vi "poc.ip.versal.vi"(0 "ip.reset":bool, 1 "TDATA":u64, 2 "TKEEP":u8, 3 "TUSER":bool, 4 "TVALID":bool, 5 "TLAST":bool) -> ()   [LabVIEW 2025]
uses:
  <vilib>/Platform/TimedLoop/XDataNode/timing_clust.ctl
  <vilib>/Platform/TimedLoop/XDataNode/nitl_modes.ctl
  <vilib>/Platform/TimedLoop/XDataNode/wakeup.ctl
  submodules/Market.Data.Common/fpga/my.network.data.stream.ctl
  submodules/Market.Data.Bats.Parser/fpga/poc.ip.debug.states.ctl
  submodules/Market.Data.Common/fpga/orderbook.command.ctl
  submodules/Market.Data.Common/fpga/orderbook.command.type.ctl
  submodules/Market.Data.Bats.Parser/fpga/poc.ip.axi.write.states.ctl
  <instrlib>/_niInstr/Network/Types/v1/IPv4 Address.ctl
  <instrlib>/_niInstr/Network/Types/v1/MAC Address.ctl
  Ethernet MAC - Custom/Ethernet MAC - Custom.lvclass
  axi_2_eth_raw.ctl
  <vilib>/rvi/DataTransferAndStorage/Container/Common/niFpgaContainerGetUniqueNameForEmu.vi
  <vilib>/rvi/DataTransferAndStorage/Container/Common/niFpgaContainerSetEmuInfo.vi
  <vilib>/rvi/eio/common/nirviEmuReportErrorAndStop.vi
  <vilib>/rvi/Emulation/niFpgaSctlEmulationGetInTimedLoop.vi
  <vilib>/rvi/Emulation/niFpgaEmulationReportErrorSimple.vi
  <vilib>/rvi/Emulation/niFpgaGetClockAttributes.vi
  <vilib>/rvi/Emulation/niFpgaCriticalErrorInLSC.vi
  <vilib>/rvi/Emulation/niFpgaEmulationIsFPGAContextNoSignature.vi
  <vilib>/rvi/errors/niFpgaSetErrorForExecOnDevCompSimple.vi
  <vilib>/rvi/FIFO/Fifo_Resource/nirvififoEmulationSetSize.vi
  <vilib>/rvi/FIFO/Fifo_Resource/nirviFifoEmulationQueueMgr.vi
  <instcachedir>/0/nirviFifoEmulationQueueMgr_E5CAEC123FF24DC58D834DCA3CDAA9B5.lvgen/nirviFifoEmulationQueueMgr_E5CAEC123FF24DC58D834DCA3CDAA9B5_002.vi
  <vilib>/Utility/error.llb/Clear Errors.vi
  <vilib>/rvi/FIFO/Fifo_Resource/nirvififoEmulationCreateLock.vi
  <vilib>/rvi/Emulation/niFpgaProcessEmulError.vi
  <vilib>/rvi/FIFO/Fifo_Resource/nirvififoEmulationObtainLock.vi
  <vilib>/rvi/FIFO/Fifo_Resource/nirvififoEmulationReleaseLock.vi
  <vilib>/rvi/occurrence/nirviWaitOnOccurrenceBase.vi
  <vilib>/rvi/errors/nirviReportUnexpectedCaseInternalError.vi
  <vilib>/rvi/errors/nirviReportUnexpectedCaseInternalError (U32).vi
  <vilib>/rvi/interface/RandomDataEmulation/nirviRandomDataMultiElementFPGAFIFO.vi
  <instcachedir>/0/nirviRandomDataMultiElementFPGAFIFO_BE2FF10D3D6E420AB0291A02835C249E.lvgen/nirviRandomDataMultiElementFPGAFIFO_BE2FF10D3D6E420AB0291A02835C249E_001.vi
  <vilib>/rvi/interface/RandomDataEmulation/niFpgaRandomDataHandleErrors.vi
  <instcachedir>/0/nirviFifoEmulationQueueMgr_E5CAEC123FF24DC58D834DCA3CDAA9B5.lvgen/nirviFifoEmulationQueueMgr_E5CAEC123FF24DC58D834DCA3CDAA9B5_004.vi
  <vilib>/rvi/DataTransferAndStorage/Container/Common/niFpgaContainerExecOnDevCompGetState.vi
  <vilib>/rvi/Memory/Memory_Emulation/niFpgaMemoryEmulationCacheClearOnFirstRun.vi
  <vilib>/rvi/Memory/Memory_Emulation/nirvimemoryEmulationManagerCache_MakeExclusive.vi
  <vilib>/rvi/Memory/Memory_Emulation/niFpgaMemoryEmulationValidateCache.vi
  <vilib>/rvi/Memory/Memory_Emulation/nirvimemoryEmulationManagerCache_InsertValue.vi
  <vilib>/rvi/Memory/Memory_Emulation/nirvimemoryEmulationManagerCache_ReleaseExclusive.vi
  <vilib>/rvi/Memory/Memory_Emulation/nirvimemoryEmulationManagerCache_GetValue.vi
  <vilib>/rvi/Memory/Memory_Emulation/nirvimemoryEmulationManagerCache_SetValue.vi
  <instcachedir>/0/nirviFifoEmulationQueueMgr_E5CAEC123FF24DC58D834DCA3CDAA9B5.lvgen/nirviFifoEmulationQueueMgr_E5CAEC123FF24DC58D834DCA3CDAA9B5_005.vi
  <vilib>/rvi/FIFO/Fifo_Resource/nirvififoEmulationDetermineInputValidOut.vi
  <vilib>/eio/utilities/niEioResolveVilibRelativePath.vi
  <instcachedir>/0/nirviFifoEmulationQueueMgr_E5CAEC123FF24DC58D834DCA3CDAA9B5.lvgen/nirviFifoEmulationQueueMgr_E5CAEC123FF24DC58D834DCA3CDAA9B5_003.vi
  <vilib>/rvi/Emulation/niFpgaSctlEmulationResourceMgr.vi
  <instrlib>/_niInstr/Network/IPv4/Data Stream/v1/Read IPv4 Header.vi
  <instrlib>/_niInstr/Network/IPv4/UDP/Data Stream/v1/Read End of Bad Frame.vi
  <instrlib>/_niInstr/Network/IPv4/UDP/Data Stream/v1/Read End of Good Frame.vi
  <instrlib>/_niInstr/Network/IPv4/UDP/Data Stream/v1/Read Data Stream.vi
  <vilib>/Platform/TimedLoop/XDataNode/XDataNode.xnode
  <vilib>/rvi/LocalResourceManager/LocalResourceManager.xnode
  <vilib>/rvi/DataTransferAndStorage/Container/XNode/niFpgaContainer.xnode
  <vilib>/rvi/FIFO/Fifo_Resource/nirvififoEmulationRead.vi
  <vilib>/rvi/interface/RandomDataEmulation/nirviRandomDataFpgaMultiElementTemplate.vi
  <vilib>/rvi/DataTransferAndStorage/Register/Emulation/niFpgaRegisterEmulationRefIn.vi
  <vilib>/rvi/FIFO/Fifo_Resource/niFpgaFifoEmulationRefIn.vi
  <vilib>/rvi/Memory/Memory_Emulation/niFpgaMemoryEmulationRefIn.vi
  <vilib>/rvi/FIFO/Fifo_Resource/nirvififoEmulationWrite.vi
  <vilib>/Platform/TimedLoop/XDataNode/XDNodeRunTimeDep.lvlib
  submodules/Market.Data.Common/fpga/fpganow.common.fpga.lvlib
  <instrlib>/_niInstr/Network/IPv4/UDP/Data Stream/v1/niInstr IPv4 UDP Data Stream v1.lvclass
  <instrlib>/_niInstr/Network/Ethernet/Utility/v1/FPGA/niInstr Ethernet Utilities FPGA v1.lvlib
  <instrlib>/_niInstr/Network/IPv4/FPGA/v1/niInstr IPv4 FPGA v1.lvlib
  <instrlib>/_niInstr/Network/IPv4/UDP/FPGA/v1/niInstr IPv4 UDP FPGA v1.lvlib
  <instrlib>/_niInstr/Network/Types/v1/niInstr Network Types v1.lvlib
  <instrlib>/_niInstr/Network/IPv4/Data Stream/v1/niInstr IPv4 Data Stream v1.lvclass
panel:
  in  "DEBUG.TREADY":bool
  in  "CMD.TREADY":bool
  in  "MDEBUG.TREADY":bool
  out "MDEBUG.TLAST":bool
  out "MDEBUG.TVALID":bool
  out "MDEBUG.TKEEP":u8
  out "MDEBUG.TDATA":u64
  out "CMD.TKEEP":u8
  out "CMD.TDATA":u64
  out "CMD.TLAST":bool
  out "CMD.TVALID":bool
  out "DEBUG.TLAST":bool
  out "DEBUG.TVALID":bool
  out "DEBUG.TKEEP":u8
  out "DEBUG.TDATA":u64
  # "This VI will be IP Exported"
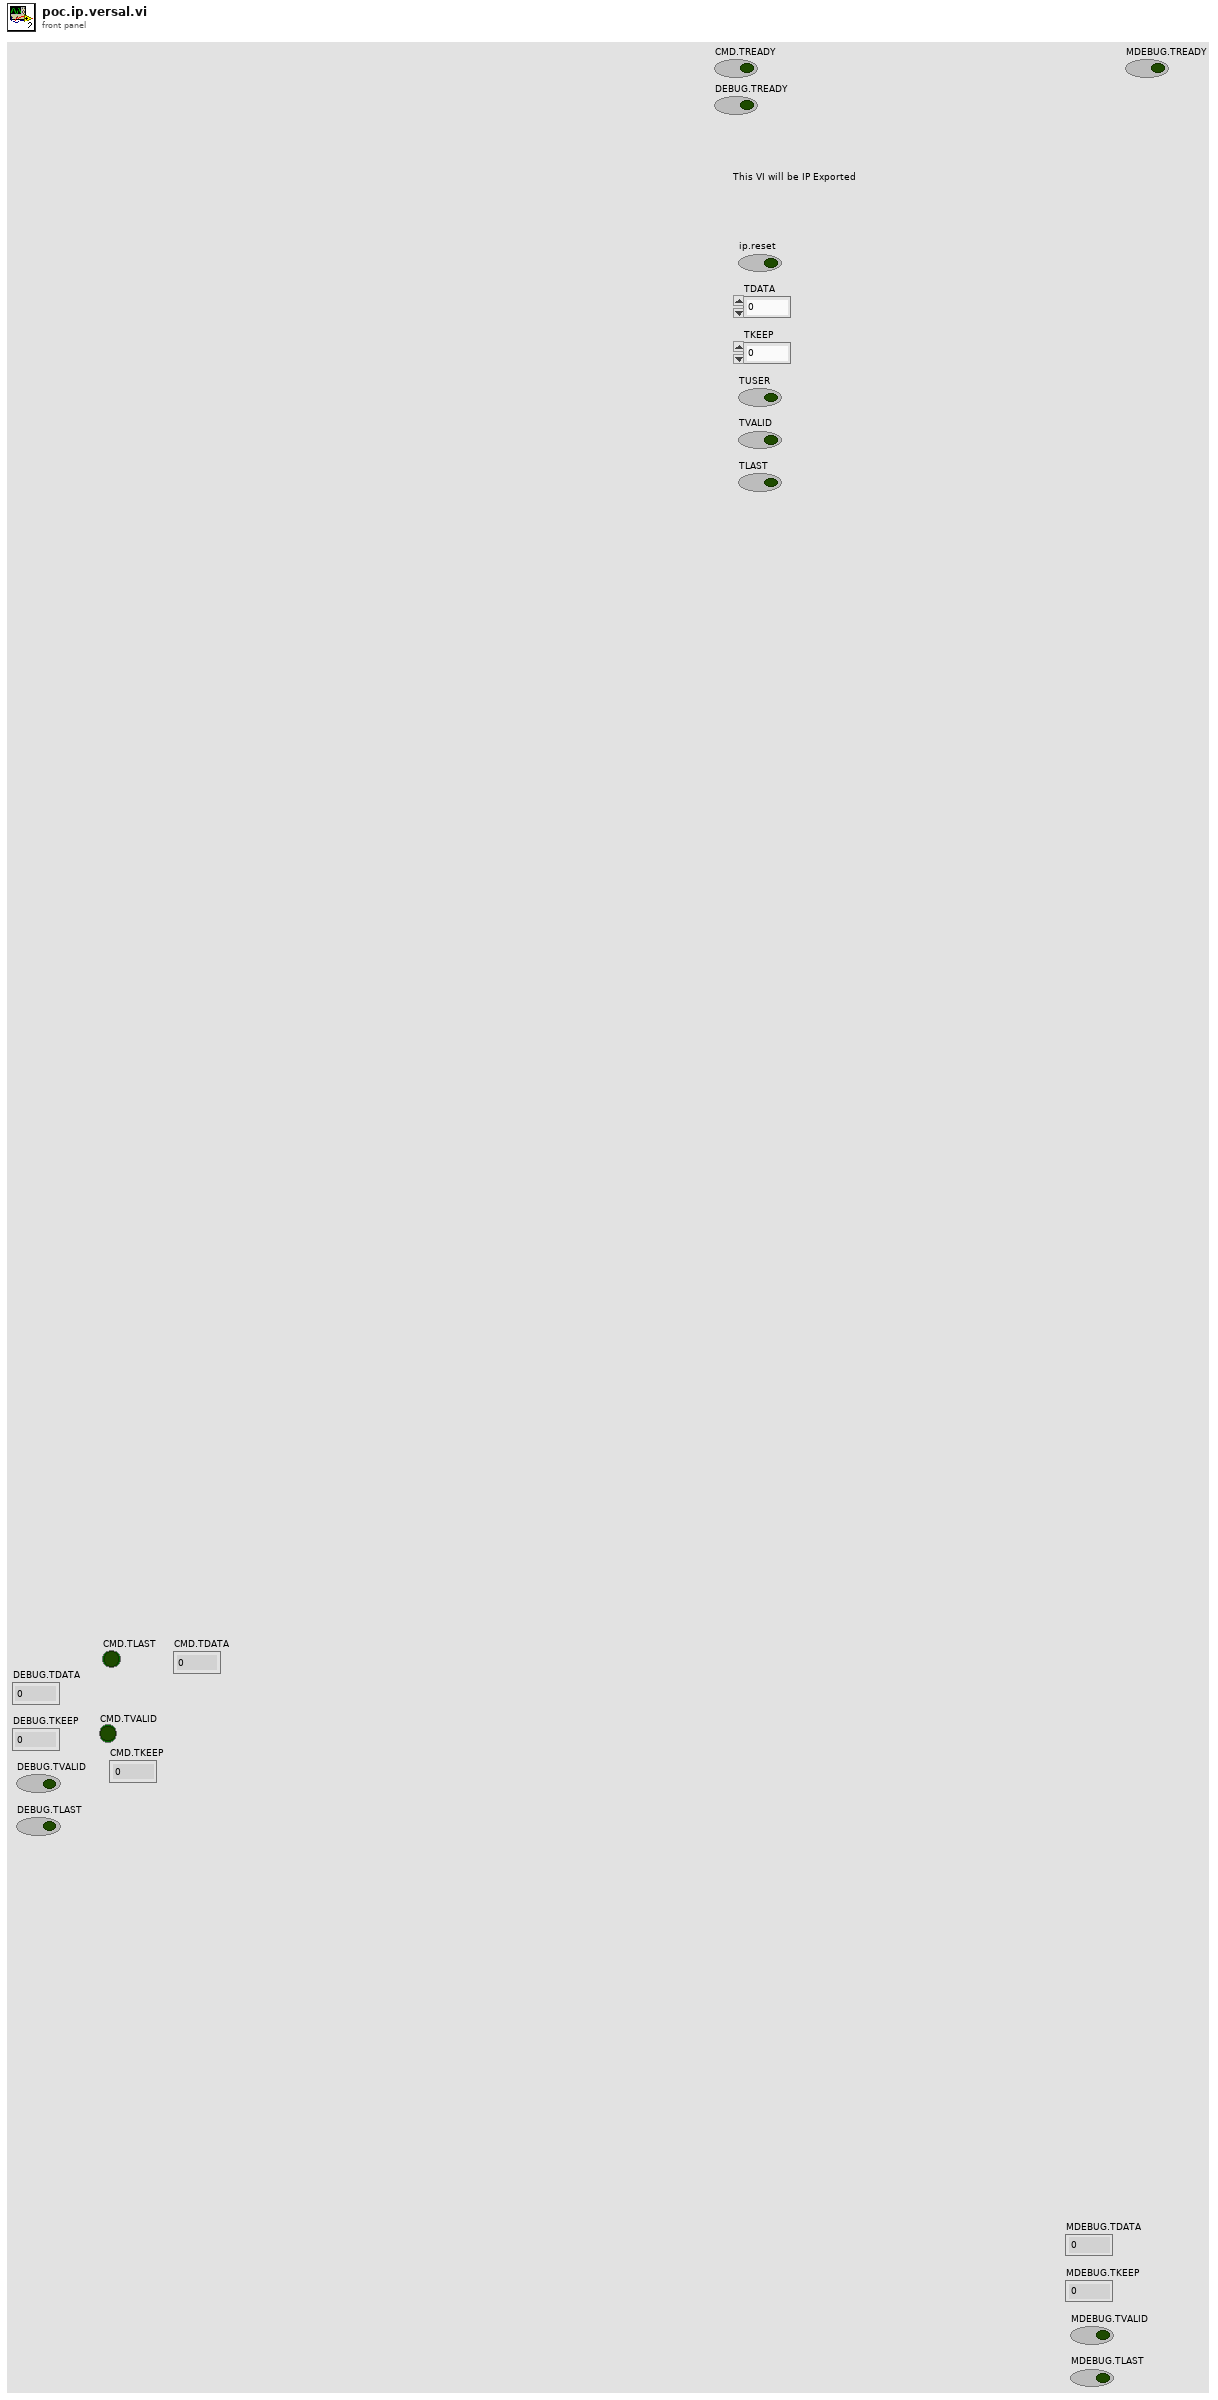
[diagram p1: front panel]
types:
  T1 = typedef "XDNodeRunTimeDep.lvlib/timing_clust.ctl" = cluster{"Expected End [f-1]":u64, "Actual End [f-1]":u64, "Finished Late? [f-1]":bool, "Expected End [i-1]":u64, "Actual End [i-1]":u64, "Finished Late? [i-1]":bool, "Expected Start [i]":u64, "Actual Start [i]":u64, "Expected Start [f]":u64, "Actual Start [f]":u64, "Source Name":string, "Structure Name":string, "Period":i64, "Deadline":i64, "Offset":i64, "Start":i64, "Priority":i32, "Timeout":i32, "Mode":T2, "Wakeup Reason":T3, "Error":errorcluster, "Source Type":string, "Secondary Source Type":string, "Global End Time":u64, "Global Start Time":u64, "Frame Duration":u64, "Iteration Duration":u64, "Assigned CPU":i32, "I/O Scan Engine Mode":u32}
  T2 = typedef "XDNodeRunTimeDep.lvlib/nitl_modes.ctl" = enum32{"No Change", "Process missed periods, maintain original phase", "Discard missed periods, maintain original phase", "Process missed periods, ignore original phase", "Discard missed periods, ignore original phase"}
  T3 = typedef "XDNodeRunTimeDep.lvlib/wakeup.ctl" = enum32{"Normal", "Aborted", "Asynchronous wakeup", "Timing source error", "Timed loop error", "Timeout"}
  T4 = typedef "niInstr Network Types v1.lvlib/MAC Address.ctl" = u8[]
  T5 = typedef "niInstr Network Types v1.lvlib/IPv4 Address.ctl" = u8[]
  T6 = typedef "my.network.data.stream.ctl" = cluster{"data":u8[], "data valid":bool, "byte enables":bool[], "eof.good":bool, "eof.bad":bool, "Timestamp":u64}
  T7 = cluster{"TDATA":u64, "TKEEP":u8, "TVALID":bool, "TLAST":bool, "TUSER":bool}
  T8 = cluster{"data valid":bool, "end.of.frame":bool, "start.of.frame":bool, "data":u64, "byte enables":u8}
  T9 = typedef "axi_2_eth_raw.ctl" = cluster{"data valid":bool, "end.of.frame":bool, "start.of.frame":bool, "data":u64, "byte enables":u8}
  T10 = typedef "niInstr IPv4 FPGA v1.lvlib/IPv4 Header.ctl" = cluster{"Version":fxp<+,4,4>, "IHL":fxp<+,4,4>, "DSCP":fxp<+,6,6>, "ECN":fxp<+,2,2>, "Total Length":u16, "Identification":u16, "Flags":fxp<+,3,3>, "Fragment Offset":fxp<+,13,13>, "Time To Live":u8, "Protocol":T11, "Header Checksum":u16, "Source IP":u8[], "Dest IP":u8[]}
  T11 = typedef "niInstr IPv4 FPGA v1.lvlib/IPv4 Protocols.ctl" = u8
  T12 = typedef "niInstr Ethernet Utilities FPGA v1.lvlib/Network Data Stream.ctl" = cluster{"data":u8[], "data valid":bool, "byte enables":bool[]}
  T13 = typedef "poc.ip.axi.write.states.ctl" = enum16{"Wait", "Collect"}
  T14 = typedef "poc.ip.debug.states.ctl" = enum16{"Wait", "Write.Data"}
  T15 = typedef "fpganow.common.fpga.lvlib/orderbook.command.ctl" = cluster{"type":T16, "side":u8, "orderId ":u64, "quantity":u32, "symbol":u64, "price":u64, "executed.qty":u32, "canceled.qty":u32, "remaining.qty":u32, "seconds":u64, "nanoseconds":u64, "Add":bool, "Edit":bool, "Remove":bool, "seq no":u32, "recv.time":u64, "parse.time":u64}
  T16 = typedef "fpganow.common.fpga.lvlib/orderbook.command.type.ctl" = enum8{"Time", "AddOrder", "OrderExecuted", "OrderExecutedAtPrice", "ReduceSize", "ModifyOrder", "DeleteOrder", "Get.Everything", "Get.All.Orders", "Get.Top"}
  T17 = cluster{"type":enum8{"Time", "AddOrder", "OrderExecuted", "OrderExecutedAtPrice", "ReduceSize", "ModifyOrder", "DeleteOrder", "Get.Everything", "Get.All.Orders", "Get.Top"}, "side":u8, "orderId ":u64, "quantity":u32, "symbol":u64, "price":u64, "executed.qty":u32, "canceled.qty":u32, "remaining.qty":u32, "seconds":u64, "nanoseconds":u64, "Add":bool, "Edit":bool, "Remove":bool, "seq no":u32, "recv.time":u64, "parse.time":u64}
  T18 = cluster{"data":u8[], "data valid":bool, "byte enables":bool[], "eof.good":bool, "eof.bad":bool, "Timestamp":u64}
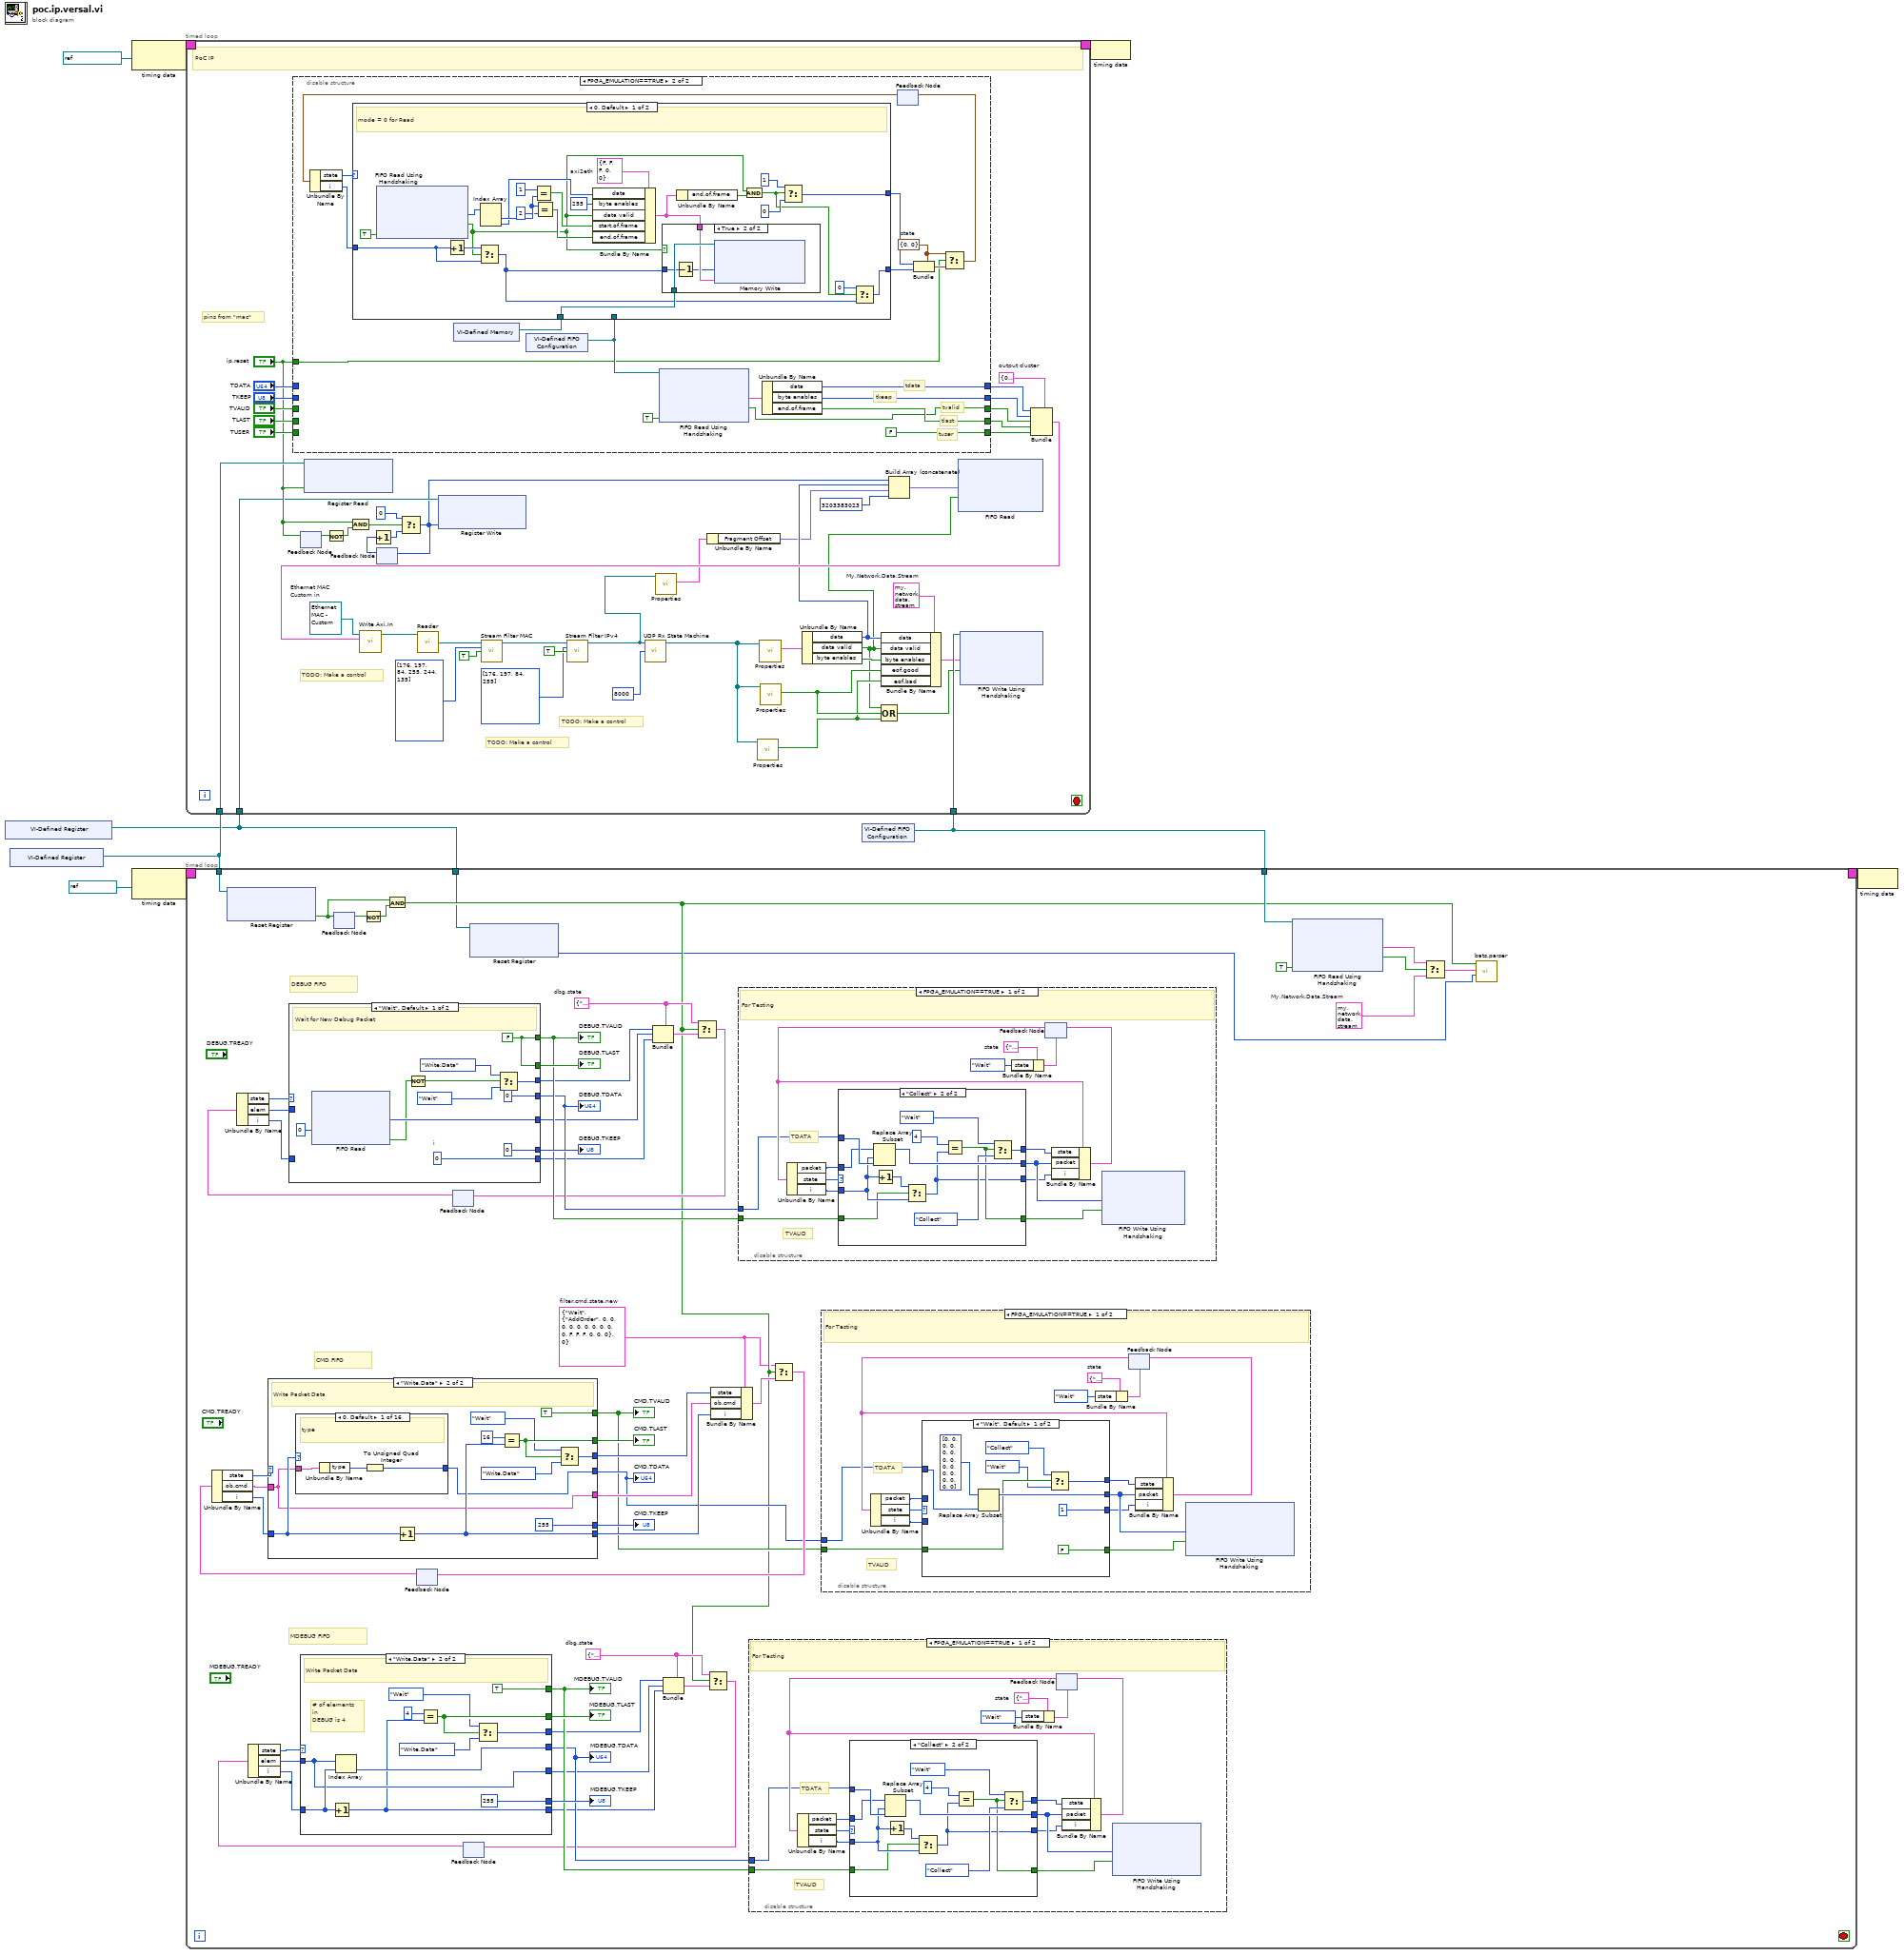
[diagram p0: block diagram]
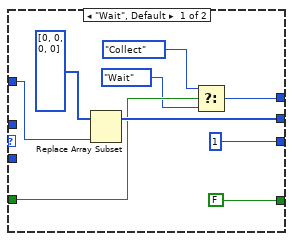
[diagram p2: hidden frame]
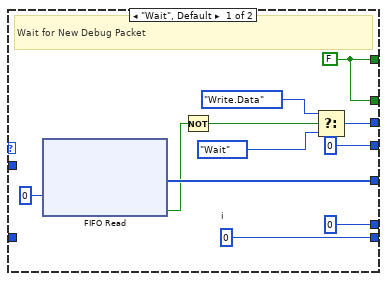
[diagram p4: hidden frame]
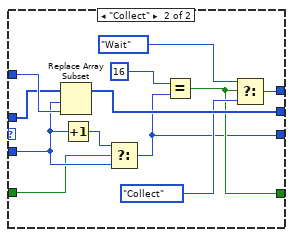
[diagram p5: hidden frame]
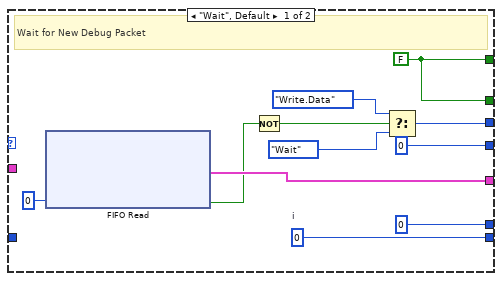
[diagram p7: hidden frame]
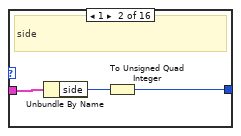
[diagram p8: hidden frame]
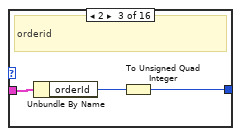
[diagram p9: hidden frame]
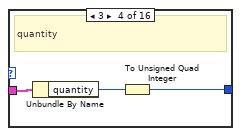
[diagram p10: hidden frame]
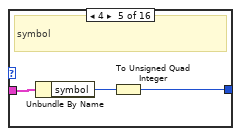
[diagram p11: hidden frame]
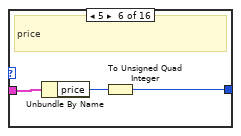
[diagram p12: hidden frame]
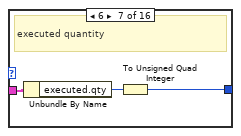
[diagram p13: hidden frame]
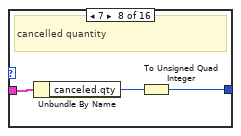
[diagram p14: hidden frame]
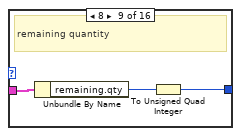
[diagram p15: hidden frame]
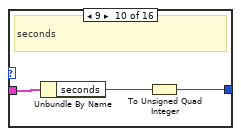
[diagram p16: hidden frame]
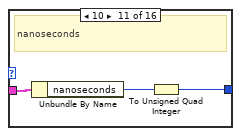
[diagram p17: hidden frame]
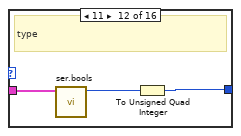
[diagram p18: hidden frame]
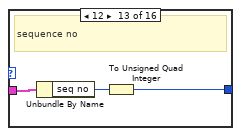
[diagram p19: hidden frame]
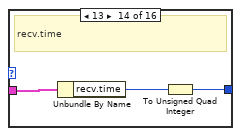
[diagram p20: hidden frame]
diagram:
  n1 = xnode "VI-Defined Register"() -> ("Register Out"=w1:refnum<k21>)
  n2 = xnode "VI-Defined Register"() -> ("Register Out"=w2:refnum<k21>)
  n3 = node-c288(refnum<k21> "156.25MHz" ("Source Name")) -> (w9:T1)
  n4 = node-c288(refnum<k21> "100MHz" ("Source Name")) -> (w6:T1)
  n5 = xnode "VI-Defined FIFO Configuration"() -> ("FIFO Out"=w3:refnum<k21>)
  n6 = timed-loop {
    timing: w9 -> [_]
    timing-out: [_] -> w8
    tunnel: w3 -> [w34]
    tunnel: w2 -> [w31]
    tunnel: w1 -> [w22]
    stop <- _ stop-if-true
    w35 = T6 {"data"=[0, 0, 0, 0, 0, 0, 0, 0], "data valid"=FALSE, "byte enables"=[FALSE, FALSE, FALSE, FALSE, FALSE, FALSE, FALSE, FALSE], "eof.good"=FALSE, "eof.bad"=FALSE, "Timestamp"=0}  # My.Network.Data.Stream
    w42 = refnum<class "Ethernet MAC - Custom.lvclass"> refnum  # Ethernet MAC Custom in
    w51 = T7 {"TDATA"=0, "TKEEP"=0, "TVALID"=FALSE, "TLAST"=FALSE, "TUSER"=FALSE}  # output cluster
    # "pins from \"mac\""
    # "TODO: Make a control"
    # "TODO: Make a control"
    # "TODO: Make a control"
    # "PoC IP"
    n7 = disable-structure shown="FPGA_EMULATION==TRUE" {
      disable-tunnel: [w61 w65] -> w41
      disable-tunnel: "TDATA" -> [w61 _]
      disable-tunnel: [w60 w64] -> w40
      disable-tunnel: "TKEEP" -> [w60 _]
      disable-tunnel: [w59 w62] -> w39
      disable-tunnel: "TVALID" -> [w59 _]
      disable-tunnel: [w58 w66] -> w38
      disable-tunnel: "TLAST" -> [w58 _]
      disable-tunnel: [w57 FALSE ("TUSER")] -> w27
      disable-tunnel: "TUSER" -> [w57 _]
      disable-tunnel: "ip.reset" -> [_ w63]
      frame condition #0 {
      }
      frame condition #1 (active) {
        w75 = cluster{"state":u8, "i":u16} {"state"=0, "i"=0}  # state
        # "tkeep"
        # "tdata"
        # "tuser"
        # "tlast"
        # "tvalid"
        n8 = xnode "VI-Defined Memory"() -> ("Memory Out"=w71:refnum<k21>)
        n9 = xnode "VI-Defined FIFO Configuration"() -> ("FIFO Out"=w68:refnum<k21>)
        n10 = xnode "FIFO Read Using Handshaking"("Ready for Output"=TRUE, "FIFO In"=w68) -> ("Element"=w69:T8, "Output Valid"=w62:bool)  [unwired: 1 out]
        n11 = Unbundle By Name(w69) -> ("data"=w65:u64, "byte enables"=w64:u8, "end.of.frame"=w66:bool)
        n12 = feedback #1() -> (w77:cluster{"state":u8, "i":u16})  [unwired: 1 in]
        n13 = Unbundle By Name(w77) -> ("state"=w78:u8, "i"=w79:u16)
        n14 = case shown="0, Default" w78 {
          tunnel: w79 -> [w91 w108]
          tunnel: w71 -> [w90 w120]
          tunnel: [w84 w114] -> w73
          tunnel: [w85 w117] -> w72
          tunnel: w68 -> [_ w107]
          frame 0, Default {
            w102 = T9 {"data valid"=FALSE, "end.of.frame"=FALSE, "start.of.frame"=FALSE, "data"=0, "byte enables"=0}  # axi2eth
            # "mode = 0 for Read"
            n15 = xnode "FIFO Read Using Handshaking"("Ready for Output"=TRUE) -> ("Element"=w101:u64[], "Output Valid"=w80:bool)  [unwired: 1 in, 1 out]
            n16 = Increment(x=w91) -> (x+1=w92:u16)
            n17 = Select(t=w92, s=w80, f=w91) -> (s? t:f=w83:u16)
            n18 = Index Array(array=w101) -> (element #1=w100:u64, element #2=w94:u64)  [unwired: 2 in]
            n19 = Equal?(x=u64 1, y=w100) -> (x = y?=w96:bool)
            n20 = Equal?(x=w100, y=u64 2) -> (x = y?=w97:bool)
            n21 = Bundle By Name(cluster=w102, "data"=w94, "byte enables"=u8 255 ("number"), "data valid"=w80, "start.of.frame"=w96, "end.of.frame"=w97) -> (w89:T9)
            n22 = case shown="True" w80 {
              tunnel: w90 -> [_ w106]
              tunnel: w89 -> [_ w105]
              tunnel: w83 -> [_ w104]
              frame False {
              }
              frame True {
                n23 = Decrement(x=w104) -> (x-1=w103:u16)
                n24 = xnode "Memory Write"("Address"=w103, "Data"=w105, "Memory In"=w106) -> ()  [unwired: 1 out]
              }
            }
            n25 = Unbundle By Name(w89) -> ("end.of.frame"=w88:bool)
            n26 = And(x=w80, y=w88) -> (x .and. y?=w82:bool)
            n27 = Select(t=u8 1, s=w82, f=u8 0 ("t")) -> (s? t:f=w85:u8)
            n28 = Select(t=u16 0, s=w82, f=w83) -> (s? t:f=w84:u16)
          }
          frame 1 {
            # "mode = 1 for Write"
            n29 = xnode "Memory Read"("Address"=w108, "Memory In"=w120) -> ("Data"=w119:T8)  [unwired: 1 out]
            n30 = feedback-in #2(w119) -> ()
            n31 = feedback #2() -> (w109:T8)  [unwired: 1 in]
            n32 = feedback-in #3(TRUE ("Input Valid")) -> ()
            n33 = feedback #3(FALSE ("Input Valid")) -> (w110:bool)
            n34 = Increment(x=w108) -> (x+1=w114:u16)
            n35 = Unbundle By Name(w109) -> ("end.of.frame"=w118:bool)
            n36 = xnode "FIFO Write Using Handshaking"("Element"=w109, "Input Valid"=w110, "FIFO In"=w107) -> ()  [unwired: 2 out]
            n37 = And(x=w118, y=w110) -> (x .and. y?=w111:bool)
            n38 = Select(t=u8 0 ("f"), s=w111, f=u8 1) -> (s? t:f=w117:u8)
          }
        }
        n39 = Bundle(cluster=w75, "state"=w72, "i"=w73) -> (w74:cluster{"state":u8, "i":u16})
        n40 = Select(t=w75, s=w63, f=w74) -> (s? t:f=w76:cluster{"state":u8, "i":u16})
        n41 = feedback-in #1(w76) -> ()
      }
    }
    n42 = feedback #4() -> (w26:bool)  [unwired: 1 in]
    n43 = feedback-in #4("ip.reset") -> ()
    n44 = xnode "Register Read"("Data"="ip.reset", "Register In"=w31) -> ()  [unwired: 1 out]
    n45 = Not(x=w26) -> (.not. x?=w25:bool)
    n46 = And(x="ip.reset", y=w25) -> (x .and. y?=w23:bool)
    n47 = feedback #5() -> (w20:u64)  [unwired: 1 in]
    n48 = Increment(x=w20) -> (x+1=w19:u64)
    n49 = Select(t=u64 0, s=w23, f=w19) -> (s? t:f=w18:u64)
    n50 = feedback-in #5(w18) -> ()
    n51 = xnode "Register Write"("Data"=w18, "Register In"=w22) -> ()  [unwired: 1 out]
    n52 = Bundle(cluster=w51, "TDATA"=w41, "TKEEP"=w40, "TVALID"=w39, "TLAST"=w38, "TUSER"=w27) -> (w37:T7)
    n53 = call-dynamic "Write Axi.In.vi"("Axi.In"=w37, "Ethernet MAC - Custom in"=w42) -> ("Ethernet MAC - Custom out"=w49:refnum<class "Ethernet MAC - Custom.lvclass">)  [unwired: 8 in, 1 out]
    n54 = call-dynamic "Reader.vi"("Ethernet MAC - Custom.lvclass"=w49) -> ("niInstr Ethernet MAC Raw Stream v1.lvclass"=w50:refnum<class "niInstr Ethernet MAC Raw Stream v1.lvclass">)  [unwired: 13 in, 1 out]
    n55 = call <instrlib>:"Stream Filter MAC.vi"("niInstr Ethernet MAC Raw Stream v1 in"=w50, "MAC Address"=T4 [176, 197, 84, 255, 244, 135], "Promiscuous?"=TRUE) -> ("niInstr Ethernet MAC Data Stream v1 out"=w43:refnum<class "niInstr Ethernet MAC Data Stream v1.lvclass">)  [unwired: 12 in]
    n56 = call <instrlib>:"Stream Filter IPv4.vi"("niInstr Ethernet MAC Data Stream v1 in"=w43, "IP Address"=T5 [176, 197, 84, 255], "disable IP filtering"=TRUE) -> ("niInstr IPv4 Data Stream out"=w13:refnum<class "niInstr IPv4 Data Stream v1.lvclass">)  [unwired: 12 in]
    n57 = call <instrlib>:"UDP Rx State Machine.vi"("niInstr IPv4 Data Stream in"=w13, "Dest Port"=u16 8000) -> ("niInstr IPv4 UDP Data Stream out"=w14:refnum<class "niInstr IPv4 UDP Data Stream v1.lvclass">)  [unwired: 13 in]
    n58 = call-poly <instrlib>:"Properties.vi"("niInstr IPv4 Data Stream in"=w13) -> ("IPv4 Header"=w12:T10)  [unwired: 9 in, 1 out]
    n59 = Unbundle By Name(w12) -> ("Fragment Offset"=w11:fxp<+,13,13>)
    n60 = call-poly <instrlib>:"Properties.vi"("niInstr IPv4 UDP Data Stream in"=w14) -> ("End of Bad Frame"=w28:bool)  [unwired: 9 in, 1 out]
    n61 = call-poly <instrlib>:"Properties.vi"("niInstr IPv4 UDP Data Stream v1.lvclass"=w14) -> ("Data Stream"=w36:T12)  [unwired: 9 in, 1 out]
    n62 = call-poly <instrlib>:"Properties.vi"("niInstr IPv4 UDP Data Stream in"=w14) -> ("End of Good Frame"=w29:bool)  [unwired: 9 in, 1 out]
    n63 = Unbundle By Name(w36) -> ("data"=w16:u8[], "data valid"=w15:bool, "byte enables"=w30:bool[])
    n64 = Bundle By Name(cluster=w35, "data"=w16, "data valid"=w15, "byte enables"=w30, "eof.good"=w29, "eof.bad"=w28) -> (w33:T6)
    n65 = Compound Arithmetic op=OR(w15, w29, w28) -> (w32:bool)
    n66 = Build Array (concatenate)(w18, w16, w11, u64 3203383023 ("element")) -> (w17:fxp<+,64,64>[])
    n67 = xnode ("FIFO Read")("Element"=w17, "Input Valid"=w15) -> ()  [unwired: 1 in, 2 out]
    n68 = xnode "FIFO Write Using Handshaking"("Element"=w33, "Input Valid"=w32, "FIFO In"=w34) -> ()  [unwired: 2 out]
  }
  n69 = timed-loop {
    timing: w6 -> [_]
    timing-out: [_] -> w5
    tunnel: w2 -> [w177]
    tunnel: w3 -> [w146]
    tunnel: w1 -> [w124]
    stop <- _ stop-if-true
    w125 = cluster{"state":T14, "ob.cmd":T15, "i":i16} {"state"=enum."Wait", "ob.cmd"={"type"=enum."AddOrder", "side"=0, "orderId "=0, "quantity"=0, "symbol"=0, "price"=0, "executed.qty"=0, "canceled.qty"=0, "remaining.qty"=0, "seconds"=0, "nanoseconds"=0, "Add"=FALSE, "Edit"=FALSE, "Remove"=FALSE, "seq no"=0, "recv.time"=0, "parse.time"=0}, "i"=0}  # filter.cmd.state.new
    w130 = cluster{"state":T14, "elem":u64[], "i":i16} {"state"=enum."Wait", "elem"=[0, 0, 0, 0], "i"=0}  # dbg.state
    w141 = T6 {"data"=[0, 0, 0, 0, 0, 0, 0, 0], "data valid"=FALSE, "byte enables"=[FALSE, FALSE, FALSE, FALSE, FALSE, FALSE, FALSE, FALSE], "eof.good"=FALSE, "eof.bad"=FALSE, "Timestamp"=0}  # My.Network.Data.Stream
    w166 = cluster{"state":T14, "elem":u64[], "i":i16} {"state"=enum."Wait", "elem"=[0, 0, 0, 0], "i"=0}  # dbg.state
    # "MDEBUG FIFO"
    # "DEBUG FIFO"
    # "CMD FIFO"
    n70 = xnode "Reset Register"("Register In"=w177) -> ("Data"=w147:bool)  [unwired: 1 out]
    n71 = feedback-in #6(w147) -> ()
    n72 = feedback #6() -> (w149:bool)  [unwired: 1 in]
    n73 = Not(x=w149) -> (.not. x?=w148:bool)
    n74 = And(x=w147, y=w148) -> (x .and. y?=w126:bool)
    n75 = feedback #7() -> (w157:cluster{"state":T14, "ob.cmd":T15, "i":i16})  [unwired: 1 in]
    n76 = Unbundle By Name(w157) -> ("state"=w156:T14, "ob.cmd"=w155:T15, "i"=w154:i16)
    n77 = case shown="\"Write.Data\"" w156 {
      tunnel: [w278 w289] -> w160
      tunnel: w154 -> [_ w283]
      tunnel: [w280 w286] -> w162
      tunnel: [w279 w282] -> w159
      tunnel: w155 -> [_ w282]
      tunnel: [u64 0 ("Data") w281] -> w151
      tunnel: [u8 0 ("DEBUG.TKEEP") u8 255 ("DEBUG.TKEEP")] -> w152
      tunnel: [w277 w287] -> w153
      tunnel: [w277 TRUE] -> w150
      frame "Wait", Default {
        w277 = FALSE
        w278 = i16 0  # i
        # "Wait for New Debug Packet"
        n78 = xnode ("FIFO Read")("Timeout"=0) -> ("Element"=w279:T17, "Timed Out?"=w270:bool)  [unwired: 1 in, 1 out]
        n79 = Not(x=w270) -> (.not. x?=w272:bool)
        n80 = Select(t=poc.ip.debug.states."Write.Data", s=w272, f=poc.ip.debug.states."Wait") -> (s? t:f=w280:T14)
      }
      frame "Write.Data" {
        # "Write Packet Data"
        n81 = case shown="0, Default" w283 {
          tunnel: w282 -> [w294 w297 w300 w303 w306 w309 w312 w315 w318 w321 w324 w327 w330 w332 w335 _]
          tunnel: [w292 w295 w298 w301 w304 w307 w310 w313 w316 w319 w322 w325 w328 w333 w336 w338] -> w281
          frame 0, Default {
            # "type"
            n82 = Unbundle By Name(w294) -> ("type"=w293:T16)
            n83 = To Unsigned Quad Integer(1:w293) -> (0:w292:u64)
          }
          frame 1 {
            # "side"
            n84 = Unbundle By Name(w297) -> ("side"=w296:u8)
            n85 = To Unsigned Quad Integer(1:w296) -> (0:w295:u64)
          }
          frame 2 {
            # "orderid"
            n86 = Unbundle By Name(w300) -> ("orderId"=w299:u64)
            n87 = To Unsigned Quad Integer(1:w299) -> (0:w298:u64)
          }
          frame 3 {
            # "quantity"
            n88 = Unbundle By Name(w303) -> ("quantity"=w302:u32)
            n89 = To Unsigned Quad Integer(1:w302) -> (0:w301:u64)
          }
          frame 4 {
            # "symbol"
            n90 = Unbundle By Name(w306) -> ("symbol"=w305:u64)
            n91 = To Unsigned Quad Integer(1:w305) -> (0:w304:u64)
          }
          frame 5 {
            # "price"
            n92 = Unbundle By Name(w309) -> ("price"=w308:u64)
            n93 = To Unsigned Quad Integer(1:w308) -> (0:w307:u64)
          }
          frame 6 {
            # "executed quantity"
            n94 = Unbundle By Name(w312) -> ("executed.qty"=w311:u32)
            n95 = To Unsigned Quad Integer(1:w311) -> (0:w310:u64)
          }
          frame 7 {
            # "cancelled quantity"
            n96 = Unbundle By Name(w315) -> ("canceled.qty"=w314:u32)
            n97 = To Unsigned Quad Integer(1:w314) -> (0:w313:u64)
          }
          frame 8 {
            # "remaining quantity"
            n98 = Unbundle By Name(w318) -> ("remaining.qty"=w317:u32)
            n99 = To Unsigned Quad Integer(1:w317) -> (0:w316:u64)
          }
          frame 9 {
            # "seconds"
            n100 = Unbundle By Name(w321) -> ("seconds"=w320:u64)
            n101 = To Unsigned Quad Integer(1:w320) -> (0:w319:u64)
          }
          frame 10 {
            # "nanoseconds"
            n102 = Unbundle By Name(w324) -> ("nanoseconds"=w323:u64)
            n103 = To Unsigned Quad Integer(1:w323) -> (0:w322:u64)
          }
          frame 11 {
            # "type"
            n104 = call "ser.bools.vi"("orderbook.command"=w327) -> ("Numeric"=w326:u32)  [unwired: 10 in]
            n105 = To Unsigned Quad Integer(1:w326) -> (0:w325:u64)
          }
          frame 12 {
            # "sequence no"
            n106 = Unbundle By Name(w330) -> ("seq no"=w329:u32)
            n107 = To Unsigned Quad Integer(1:w329) -> (0:w328:u64)
          }
          frame 13 {
            # "recv.time"
            n108 = Unbundle By Name(w332) -> ("recv.time"=w331:u64)
            n109 = To Unsigned Quad Integer(1:w331) -> (0:w333:u64)
          }
          frame 14 {
            # "parse.time"
            n110 = Unbundle By Name(w335) -> ("parse.time"=w334:u64)
            n111 = To Unsigned Quad Integer(1:w334) -> (0:w336:u64)
          }
          frame 15 {
            # "Reserved for Filter time"
            n112 = To Unsigned Quad Integer(1:u64 3735928559 ("number")) -> (0:w338:u64)
          }
        }
        n113 = Increment(x=w283) -> (x+1=w289:i16)
        n114 = Equal?(x=i16 16, y=w289) -> (x = y?=w287:bool)
        n115 = Select(t=poc.ip.debug.states."Wait", s=w287, f=poc.ip.debug.states."Write.Data") -> (s? t:f=w286:T14)
      }
    }
    "CMD.TVALID" <- w150
    "CMD.TLAST" <- w153
    "CMD.TDATA" <- w151
    "CMD.TKEEP" <- w152
    n116 = feedback #8() -> (w167:cluster{"state":T14, "elem":u64[], "i":i16})  [unwired: 1 in]
    n117 = Unbundle By Name(w167) -> ("state"=w165:T14, "elem"=w164:u64[], "i"=w163:i16)
    n118 = case shown="\"Wait\", Default" w165 {
      tunnel: [w382 w390] -> w170
      tunnel: w163 -> [_ w395]
      tunnel: [w384 w387] -> w172
      tunnel: [w383 w394] -> w171
      tunnel: w164 -> [_ w394]
      tunnel: [u64 0 ("Data") w393] -> w173
      tunnel: [u8 0 ("DEBUG.TKEEP") u8 255 ("DEBUG.TKEEP")] -> w176
      tunnel: [w381 w388] -> w175
      tunnel: [w381 TRUE] -> w174
      frame "Wait", Default {
        w381 = FALSE
        w382 = i16 0  # i
        # "Wait for New Debug Packet"
        n119 = xnode ("FIFO Read")("Timeout"=0) -> ("Element"=w383:u64[], "Timed Out?"=w374:bool)  [unwired: 1 in, 1 out]
        n120 = Not(x=w374) -> (.not. x?=w376:bool)
        n121 = Select(t=poc.ip.debug.states."Write.Data", s=w376, f=poc.ip.debug.states."Wait") -> (s? t:f=w384:T14)
      }
      frame "Write.Data" {
        # "# of elements \nin \nDEBUG is 4"
        # "Write Packet Data"
        n122 = Increment(x=w395) -> (x+1=w390:i16)
        n123 = Index Array(array=w394, index=w395) -> (element=w393:u64)
        n124 = Equal?(x=i16 4, y=w390) -> (x = y?=w388:bool)
        n125 = Select(t=poc.ip.debug.states."Wait", s=w388, f=poc.ip.debug.states."Write.Data") -> (s? t:f=w387:T14)
      }
    }
    "DEBUG.TDATA" <- w173
    "DEBUG.TKEEP" <- w176
    "DEBUG.TVALID" <- w174
    "DEBUG.TLAST" <- w175
    n126 = feedback #9() -> (w131:cluster{"state":T14, "elem":u64[], "i":i16})  [unwired: 1 in]
    n127 = Unbundle By Name(w131) -> ("state"=w129:T14, "elem"=w128:u64[], "i"=w127:i16)
    n128 = case shown="\"Write.Data\"" w129 {
      tunnel: [w221 w229] -> w134
      tunnel: w127 -> [_ w234]
      tunnel: [w223 w226] -> w136
      tunnel: [w222 w233] -> w135
      tunnel: w128 -> [_ w233]
      tunnel: [u64 0 ("Data") w232] -> w137
      tunnel: [u8 0 ("DEBUG.TKEEP") u8 255 ("DEBUG.TKEEP")] -> w140
      tunnel: [w220 w227] -> w139
      tunnel: [w220 TRUE] -> w138
      frame "Wait", Default {
        w220 = FALSE
        w221 = i16 0  # i
        # "Wait for New Debug Packet"
        n129 = xnode ("FIFO Read")("Timeout"=0) -> ("Element"=w222:u64[], "Timed Out?"=w213:bool)  [unwired: 1 in, 1 out]
        n130 = Not(x=w213) -> (.not. x?=w215:bool)
        n131 = Select(t=poc.ip.debug.states."Write.Data", s=w215, f=poc.ip.debug.states."Wait") -> (s? t:f=w223:T14)
      }
      frame "Write.Data" {
        # "# of elements \nin \nDEBUG is 4"
        # "Write Packet Data"
        n132 = Increment(x=w234) -> (x+1=w229:i16)
        n133 = Index Array(array=w233, index=w234) -> (element=w232:u64)
        n134 = Equal?(x=i16 4, y=w229) -> (x = y?=w227:bool)
        n135 = Select(t=poc.ip.debug.states."Wait", s=w227, f=poc.ip.debug.states."Write.Data") -> (s? t:f=w226:T14)
      }
    }
    "MDEBUG.TDATA" <- w137
    "MDEBUG.TKEEP" <- w140
    "MDEBUG.TVALID" <- w138
    "MDEBUG.TLAST" <- w139
    n136 = xnode "Reset Register"("Register In"=w124) -> ("Data"=w123:u64)  [unwired: 1 out]
    n137 = Bundle(cluster=w166, "state"=w172, "elem"=w171, "i"=w170) -> (w169:cluster{"state":T14, "elem":u64[], "i":i16})
    n138 = Bundle(cluster=w130, "state"=w136, "elem"=w135, "i"=w134) -> (w133:cluster{"state":T14, "elem":u64[], "i":i16})
    n139 = Select(t=w166, s=w126, f=w169) -> (s? t:f=w168:cluster{"state":T14, "elem":u64[], "i":i16})
    n140 = feedback-in #8(w168) -> ()
    n141 = Select(t=w130, s=w126, f=w133) -> (s? t:f=w132:cluster{"state":T14, "elem":u64[], "i":i16})
    n142 = feedback-in #9(w132) -> ()
    n143 = Bundle By Name(cluster=w125, "state"=w162, "ob.cmd"=w159, "i"=w160) -> (w161:cluster{"state":T14, "ob.cmd":T15, "i":i16})
    n144 = disable-structure shown="FPGA_EMULATION==TRUE" {
      disable-tunnel: w174 -> [w340 _]
      disable-tunnel: w173 -> [w339 _]
      frame condition #0 (active) {
        w341 = cluster{"state":T13, "packet":u64[], "i":u16} {"state"=enum."Wait", "packet"=[0, 0, 0, 0], "i"=0}  # state
        # "TVALID"
        # "TDATA"
        # "For Testing"
        n145 = Bundle By Name(cluster=w341, "state"=poc.ip.axi.write.states."Wait" ("Enum")) -> (w345:cluster{"state":T13, "packet":u64[], "i":u16})
        n146 = feedback #10(w345) -> (w346:cluster{"state":T13, "packet":u64[], "i":u16})
        n147 = Unbundle By Name(w346) -> ("packet"=w351:u64[], "state"=w342:T13, "i"=w350:u16)
        n148 = case shown="\"Collect\"" w342 {
          tunnel: [FALSE w367] -> w343
          tunnel: [w353 w366] -> w348
          tunnel: w340 -> [w355 w363]
          tunnel: w339 -> [w358 w373]
          tunnel: [u16 1 ("i") w362] -> w349
          tunnel: [w357 w371] -> w352
          tunnel: w350 -> [_ w364]
          tunnel: w351 -> [_ w372]
          frame "Wait", Default {
            n149 = Replace Array Subset(array=u64[] [0, 0, 0, 0] ("packet"), new element=w358) -> (w357:u64[])  [unwired: 1 in]
            n150 = Select(t=poc.ip.axi.write.states."Collect" ("state"), s=w355, f=poc.ip.axi.write.states."Wait" ("state")) -> (s? t:f=w353:T13)
          }
          frame "Collect" {
            n151 = Replace Array Subset(array=w372, new element=w373, index=w364) -> (w371:u64[])
            n152 = Increment(x=w364) -> (x+1=w365:u16)
            n153 = Select(t=w365, s=w363, f=w364) -> (s? t:f=w362:u16)
            n154 = Equal?(x=u16 4, y=w362) -> (x = y?=w367:bool)
            n155 = Select(t=poc.ip.axi.write.states."Wait" ("Enum"), s=w367, f=poc.ip.axi.write.states."Collect" ("Enum")) -> (s? t:f=w366:T13)
          }
        }
        n156 = Bundle By Name(cluster=w346, "state"=w348, "packet"=w352, "i"=w349) -> (w347:cluster{"state":T13, "packet":u64[], "i":u16})
        n157 = feedback-in #10(w347) -> ()
        n158 = xnode "FIFO Write Using Handshaking"("Element"=w352, "Input Valid"=w343) -> ()  [unwired: 1 in, 2 out]
      }
      frame condition #1 {
      }
    }
    n159 = disable-structure shown="FPGA_EMULATION==TRUE" {
      disable-tunnel: w138 -> [w179 _]
      disable-tunnel: w137 -> [w178 _]
      frame condition #0 (active) {
        w180 = cluster{"state":T13, "packet":u64[], "i":u16} {"state"=enum."Wait", "packet"=[0, 0, 0, 0], "i"=0}  # state
        # "TVALID"
        # "TDATA"
        # "For Testing"
        n160 = Bundle By Name(cluster=w180, "state"=poc.ip.axi.write.states."Wait" ("Enum")) -> (w184:cluster{"state":T13, "packet":u64[], "i":u16})
        n161 = feedback #11(w184) -> (w185:cluster{"state":T13, "packet":u64[], "i":u16})
        n162 = Unbundle By Name(w185) -> ("packet"=w190:u64[], "state"=w181:T13, "i"=w189:u16)
        n163 = case shown="\"Collect\"" w181 {
          tunnel: [FALSE w206] -> w182
          tunnel: [w192 w205] -> w187
          tunnel: w179 -> [w194 w202]
          tunnel: w178 -> [w197 w212]
          tunnel: [u16 1 ("i") w201] -> w188
          tunnel: [w196 w210] -> w191
          tunnel: w189 -> [_ w203]
          tunnel: w190 -> [_ w211]
          frame "Wait", Default {
            n164 = Replace Array Subset(array=u64[] [0, 0, 0, 0] ("packet"), new element=w197) -> (w196:u64[])  [unwired: 1 in]
            n165 = Select(t=poc.ip.axi.write.states."Collect" ("state"), s=w194, f=poc.ip.axi.write.states."Wait" ("state")) -> (s? t:f=w192:T13)
          }
          frame "Collect" {
            n166 = Replace Array Subset(array=w211, new element=w212, index=w203) -> (w210:u64[])
            n167 = Increment(x=w203) -> (x+1=w204:u16)
            n168 = Select(t=w204, s=w202, f=w203) -> (s? t:f=w201:u16)
            n169 = Equal?(x=u16 4, y=w201) -> (x = y?=w206:bool)
            n170 = Select(t=poc.ip.axi.write.states."Wait" ("Enum"), s=w206, f=poc.ip.axi.write.states."Collect" ("Enum")) -> (s? t:f=w205:T13)
          }
        }
        n171 = Bundle By Name(cluster=w185, "state"=w187, "packet"=w191, "i"=w188) -> (w186:cluster{"state":T13, "packet":u64[], "i":u16})
        n172 = feedback-in #11(w186) -> ()
        n173 = xnode "FIFO Write Using Handshaking"("Element"=w191, "Input Valid"=w182) -> ()  [unwired: 1 in, 2 out]
      }
      frame condition #1 {
      }
    }
    n174 = Select(t=w125, s=w126, f=w161) -> (s? t:f=w158:cluster{"state":T14, "ob.cmd":T15, "i":i16})
    n175 = feedback-in #7(w158) -> ()
    n176 = disable-structure shown="FPGA_EMULATION==TRUE" {
      disable-tunnel: w150 -> [w236 _]
      disable-tunnel: w151 -> [w235 _]
      frame condition #0 (active) {
        w237 = cluster{"state":T13, "packet":u64[], "i":u16} {"state"=enum."Wait", "packet"=[0, 0, 0, 0, 0, 0, 0, 0, 0, 0, 0, 0, 0, 0, 0, 0], "i"=0}  # state
        # "TVALID"
        # "TDATA"
        # "For Testing"
        n177 = Bundle By Name(cluster=w237, "state"=poc.ip.axi.write.states."Wait" ("Enum")) -> (w241:cluster{"state":T13, "packet":u64[], "i":u16})
        n178 = feedback #12(w241) -> (w242:cluster{"state":T13, "packet":u64[], "i":u16})
        n179 = Unbundle By Name(w242) -> ("packet"=w247:u64[], "state"=w238:T13, "i"=w246:u16)
        n180 = case shown="\"Wait\", Default" w238 {
          tunnel: [FALSE w263] -> w239
          tunnel: [w249 w262] -> w244
          tunnel: w236 -> [w251 w259]
          tunnel: w235 -> [w254 w269]
          tunnel: [u16 1 ("i") w258] -> w245
          tunnel: [w253 w267] -> w248
          tunnel: w246 -> [_ w260]
          tunnel: w247 -> [_ w268]
          frame "Wait", Default {
            n181 = Replace Array Subset(array=u64[] [0, 0, 0, 0, 0, 0, 0, 0, 0, 0, 0, 0, 0, 0, 0, 0] ("packet"), new element=w254) -> (w253:u64[])  [unwired: 1 in]
            n182 = Select(t=poc.ip.axi.write.states."Collect" ("state"), s=w251, f=poc.ip.axi.write.states."Wait" ("state")) -> (s? t:f=w249:T13)
          }
          frame "Collect" {
            n183 = Replace Array Subset(array=w268, new element=w269, index=w260) -> (w267:u64[])
            n184 = Increment(x=w260) -> (x+1=w261:u16)
            n185 = Select(t=w261, s=w259, f=w260) -> (s? t:f=w258:u16)
            n186 = Equal?(x=u16 16, y=w258) -> (x = y?=w263:bool)
            n187 = Select(t=poc.ip.axi.write.states."Wait" ("Enum"), s=w263, f=poc.ip.axi.write.states."Collect" ("Enum")) -> (s? t:f=w262:T13)
          }
        }
        n188 = Bundle By Name(cluster=w242, "state"=w244, "packet"=w248, "i"=w245) -> (w243:cluster{"state":T13, "packet":u64[], "i":u16})
        n189 = feedback-in #12(w243) -> ()
        n190 = xnode "FIFO Write Using Handshaking"("Element"=w248, "Input Valid"=w239) -> ()  [unwired: 1 in, 2 out]
      }
      frame condition #1 {
      }
    }
    n191 = xnode "FIFO Read Using Handshaking"("Ready for Output"=TRUE, "FIFO In"=w146) -> ("Element"=w143:T18, "Output Valid"=w144:bool)  [unwired: 1 out]
    n192 = Select(t=w143, s=w144, f=w141) -> (s? t:f=w142:T6)
    n193 = call "bats.parser.vi"("time"=w123, "data.stream"=w142, "reset"=w126) -> ()  [unwired: 8 in, 1 out]
  }
  n194 = node-c288(w8) -> ()
  n195 = node-c288(w5) -> ()
